vi "Get subunit.vi"(8 "error in (no error)":errorcluster, 11 "PIPXI40 Base in":refnum<class "PIPXI40 Base.lvclass">) -> (0 "error out":errorcluster, 2 "subunit":u32=1, 3 "PIPXI40 Base out":refnum<class "PIPXI40 Base.lvclass">)   [LabVIEW 2020, in "PIPXI40.lvlib" / "PIPXI40 Base.lvclass"]
uses:
  PIPXI40 Base.lvclass
  PIPXI40 Base.lvclass/PIPXI40 Base.ctl
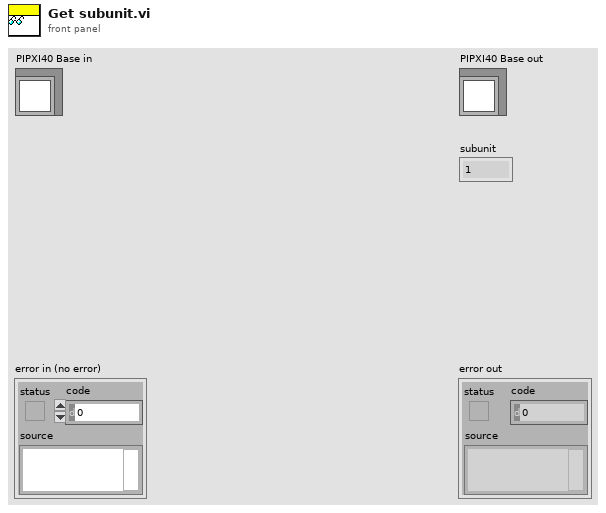
[diagram p1: front panel]
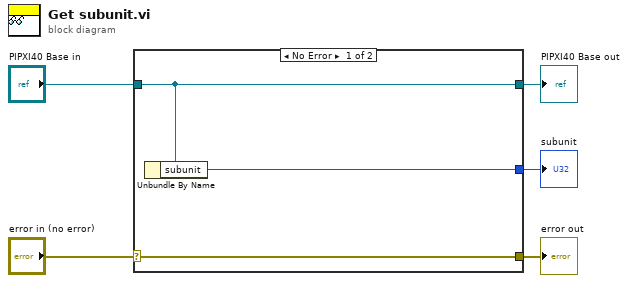
[diagram p0: block diagram]
diagram:
  n1 = case shown="No Error" "error in (no error)" {
    selector: "error in (no error)" -> [w8 w9]
    tunnel: [w8 w9] -> w4
    tunnel: [w7 w10] -> w2
    tunnel: "PIPXI40 Base in" -> [w7 w10]
    tunnel: [w6 _] -> w1
    frame No Error {
      n2 = Unbundle By Name(w7) -> ("subunit"=w6:u32)
    }
    frame Error {
    }
  }
  "error out" <- w4
  "PIPXI40 Base out" <- w2
  "subunit" <- w1
